vi "Handle Request Error.vi"(8 "error in (no error)":errorcluster, 10 "Response":T1) -> (0 "error out":errorcluster)   [LabVIEW 2015, in "NI_Azure_Queue.lvlib"]
uses:
  NI_Azure_Queue.lvlib
  Core/Response.ctl
  Core/NI_Azure_Core.lvlib
  XML Parsing/NI_Azure_XML Parsing.lvlib
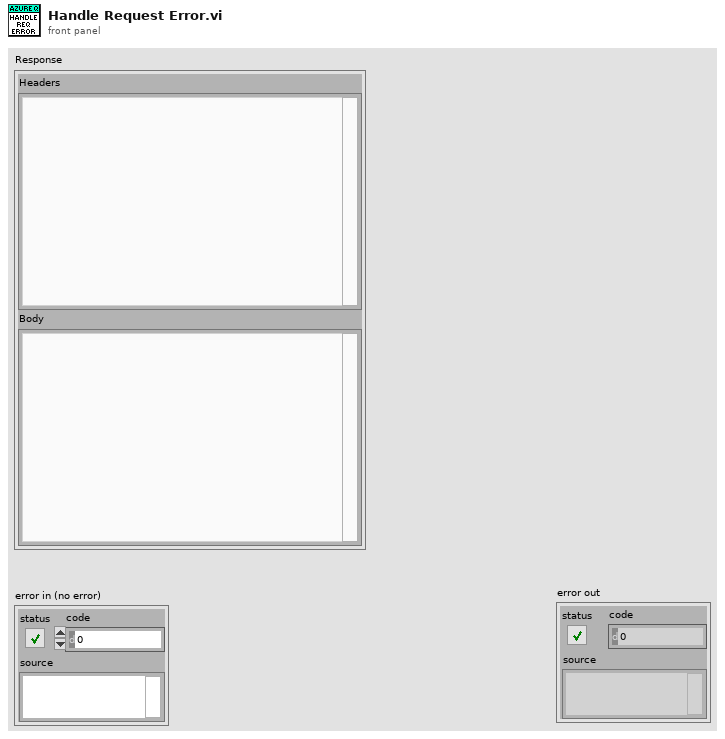
[diagram p1: front panel]
types:
  T1 = typedef "NI_Azure_Core.lvlib/Response.ctl" = cluster{"Headers":string, "Body":string}
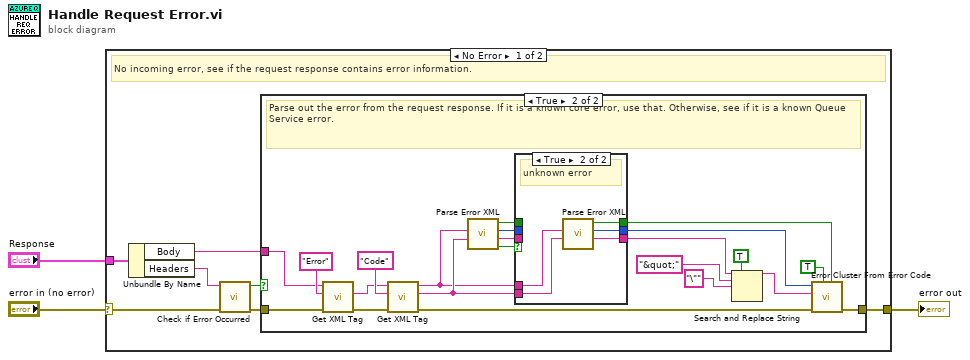
[diagram p0: block diagram]
diagram:
  n1 = case shown="No Error" "error in (no error)" {
    selector: "error in (no error)" -> [w10 w42]
    tunnel: [w5 w42] -> w2
    tunnel: "Response" -> [w9 _]
    frame No Error {
      # "No incoming error, see if the request response contains error information."
      n2 = Unbundle By Name(w9) -> ("Body"=w4:string, "Headers"=w8:string)
      n3 = call "Check if Error Occurred.vi"("error in (no error)"=w10, "Response header"=w8) -> ("error out"=w6:errorcluster, "Error Occurred"=w7:bool)  [unwired: 8 in]
      n4 = case shown="True" w7 {
        tunnel: w6 -> [w11 w29]
        tunnel: [w11 w23] -> w5
        tunnel: w4 -> [_ w28]
        frame False {
          # "No error in the request response."
        }
        frame True {
          # "Parse out the error from the request response. If it is a known core error, use that. Otherwise, see if it is a known Queue Service error."
          n5 = call "Get XML Tag.vi"("error in (no error)"=w29, "Tag name"="Error", "XML String in"=w28) -> ("error out"=w31:errorcluster, "Tag value"=w32:string)  [unwired: 4 in, 3 out]
          n6 = call "Get XML Tag.vi"("error in (no error)"=w31, "Tag name"="Code", "XML String in"=w32) -> ("error out"=w22:errorcluster, "Tag value"=w20:string, "XML String dup"=w19:string)  [unwired: 4 in, 2 out]
          n7 = call "Parse Error XML.vi"("Code Tag Value"=w20, "Error XML"=w19) -> ("Unknown Error"=w27:bool, "Error Description Override"=w24:string, "Error Code"=w25:i32, "Warning"=w26:bool)  [unwired: 6 in]
          n8 = case shown="True" w27 {
            tunnel: w26 -> [w36 _]
            tunnel: w25 -> [w35 _]
            tunnel: w24 -> [w34 _]
            tunnel: [w36 w41] -> w17
            tunnel: [w35 w40] -> w18
            tunnel: [w34 w39] -> w13
            tunnel: w20 -> [_ w37]
            tunnel: w19 -> [_ w38]
            frame False {
              # "known core error"
            }
            frame True {
              # "unknown error"
              n9 = call "Parse Error XML.vi"("Code Tag Value"=w37, "Error XML"=w38) -> ("Error Description Override"=w39:string, "Error Code"=w40:i32, "Warning"=w41:bool)  [unwired: 6 in, 1 out]
            }
          }
          n10 = Search and Replace String(replace all?=TRUE ("replace all? (F)"), input string=w13, search string="&quot;", replace string="\"") -> (result string=w12:string)  [unwired: 4 in, 3 out]
          n11 = call <vilib>:"Error Cluster From Error Code.vi"("is warning? (False)"=w17, "show call chain? (False)"=TRUE, "error in (no error)"=w22, "error message (\"\")"=w12, "error code (0)"=w18) -> ("error out"=w23:errorcluster)  [unwired: 4 in]
        }
      }
    }
    frame Error {
      # "Incoming error, do not modify the error stream."
    }
  }
  "error out" <- w2
